vi "Read Multiple Digital Inputs and Get High Times.vi"(0 "Lines":tag, 5 "Rate (Hz)":dbl=1000.0 format="%0.2f", 7 "Samples":i32=1000, 11 "Error In":errorcluster) -> (4 "High Times (s)":dbl[][](array[numeric])=[[0.048, 19.932000000000002, 0.0], [0.256, 9.626, 10.098], [0.254, 9.628, 10.098], [0.256, 9.625, 10.099], [0.047, 19.933, 0.0], [0.253, 10.701, 9.026], [0.255, 10.699, 9.026], [0.048, 19.932000000000002, 0.0], [0.258, 8.014, 11.708], [0.256, 8.016, 11.708], [0.256, 8.016, 11.708], [0.048, 19.932000000000002, 0.0], [0.254, 7.527, 12.199], [0.047, 19.933, 0.0], [0.253, 6.848, 12.879]], 15 "Error Out":errorcluster)   [LabVIEW 2016]
doc: "This VI reads multiple digital input lines and provides an array output of high/low times."
uses:
  <vilib>/DAQmx/read.llb/DAQmx Read (Digital 1D Wfm NChan NSamp).vi
  <vilib>/DAQmx/create/channels.llb/DAQmx Create Channel (DI-Digital Input).vi
  <vilib>/DAQmx/configure/timing.llb/DAQmx Timing (Sample Clock).vi
  <vilib>/DAQmx/miscellaneous.llb/DAQmx Fill In Error Info.vi
panel:
  out "Digital Waveform Graph":digitalwaveform[](graph)
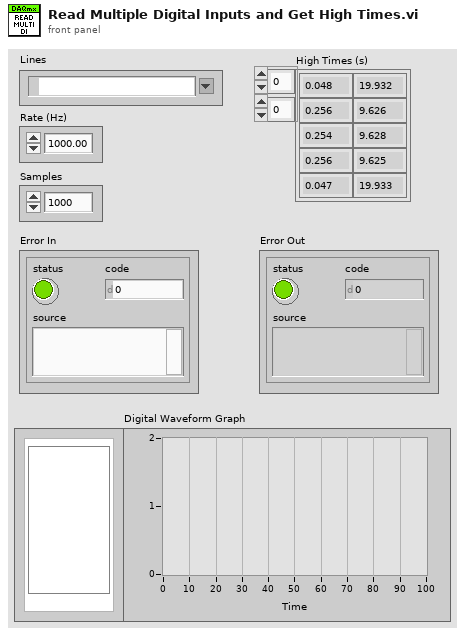
[diagram p1: front panel]
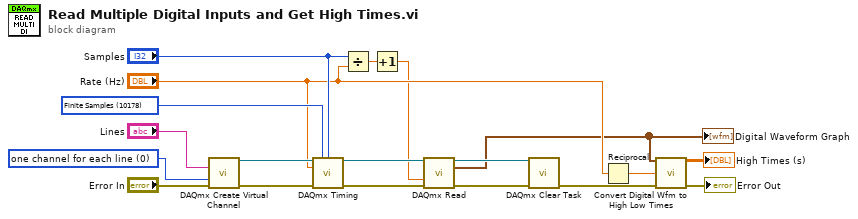
[diagram p0: block diagram]
diagram:
  w10 = 10178 items=["Finite Samples"=10178, "Continuous Samples"=10123, "Hardware Timed Single Point"=12522] ("sample mode")
  w19 = 0 items=["one channel for each line", "one channel for all lines"] ("line grouping")
  n1 = call-poly <vilib>:"DAQmx Create Virtual Channel.vi"("lines"="Lines", "line grouping"=w19, "error in"="Error In") -> ("task out"=w14:refnum<k21>, "error out"=w13:errorcluster)  [unwired: 11 in]
  n2 = call-poly <vilib>:"DAQmx Timing.vi"("task/channels in"=w14, "sample mode"=w10, "samples per channel"="Samples", "rate"="Rate (Hz)", "error in"=w13) -> ("task out"=w12:refnum<k21>, "error out"=w11:errorcluster)  [unwired: 9 in]
  n3 = Divide(x="Samples", y="Rate (Hz)") -> (x/y=w4:dbl)
  n4 = Increment(x=w4) -> (x+1=w3:dbl)
  n5 = call-poly <vilib>:"DAQmx Read.vi"("task/channels in"=w12, "timeout"=w3, "error in"=w11) -> ("task out"=w17:refnum<k21>, "data"=w1:digitalwaveform[], "error out"=w18:errorcluster)  [unwired: 10 in]
  "Digital Waveform Graph" <- w1
  n6 = call <vilib>:"DAQmx Clear Task.vi"("task in"=w17, "error in"=w18) -> ("error out"=w8:errorcluster)  [unwired: 13 in]
  n7 = Reciprocal(x="Rate (Hz)") -> (1/x=w9:dbl)
  n8 = call "Convert Digital Wfm to High Low Times.vi"("Digital Waveform In"=w1, "Dt"=w9, "Error In"=w8) -> ("HL Raw Output"=→"High Times (s)":dbl[][], "Error Out"=→"Error Out":errorcluster)  [unwired: 11 in]
